vi "h5_data_2D.vi"(8 "error in (no error)":errorcluster, 11 "data":T1={"files"=[], "record"=FALSE, "save traces"=FALSE, "raw data"=[], "scope_position"=0.0, "cursors"={"A"=0.0, "B"=0.0, "C"=0.0, "D"=0.0, "E"=0.0, "F"=0.0}, "analysis_result"={"v0"=0.0, "v1"=0.0, "w0"=0.0, "w1"=0.0, "a0"=0.0, "a1"=0.0, "a2"=0.0, "f"=0.0}, "analysis_pars"=[], "func"="a0 - a1"}) -> (0 "error out":errorcluster)   [LabVIEW 2017, in "tools.lvlib"]
uses:
  tools.lvlib
  data_2D.ctl
  analysis/cursors.ctl
  analysis/analysis_result2D.ctl
  analysis/analysis_parameters.ctl
  <vilib>/UPVI/lvhdf5/dataset.llb/LVH5D Operation.ctl
  <vilib>/UPVI/lvhdf5/file.llb/LVH5F Operation.ctl
  <vilib>/UPVI/lvhdf5/dataset.llb/Simple OpenCreateReplace Dataset (Variant).vi
  <vilib>/Utility/VariantDataType/GetClusterInfo.vi
  <vilib>/Utility/VariantDataType/GetTypeInfo.vi
  <vilib>/UPVI/lvhdf5/attribute.llb/Write Multiple Attributes.vi
  <vilib>/UPVI/lvhdf5/attribute.llb/Simple H5Awrite (Variant).vi
  <vilib>/UPVI/lvhdf5/dataset.llb/H5Dwrite (Variant).vi
  <vilib>/UPVI/lvhdf5/dataset.llb/Append Element(s) to Dataset (Variant).vi
  <vilib>/UPVI/lvhdf5/dataset.llb/Simple OpenCreateReplace Dataset.xnode
  <vilib>/UPVI/lvhdf5/library.llb/HDF5 Ref.ctl
  <vilib>/UPVI/lvhdf5/attribute.llb/LVH5A Operation.ctl
  <vilib>/UPVI/lvhdf5/attribute.llb/LVH5 Write Attributes.xnode
  <vilib>/UPVI/lvhdf5/attribute.llb/Cluster to Attribute Array.xnode
  <vilib>/UPVI/lvhdf5/attribute.llb/Simple H5Awrite.xnode
  <vilib>/UPVI/lvhdf5/dataset.llb/H5Dwrite.xnode
  <vilib>/UPVI/lvhdf5/dataset.llb/Append Element(s) to Dataset.xnode
  <vilib>/Utility/VariantDataType/VariantType.lvlib
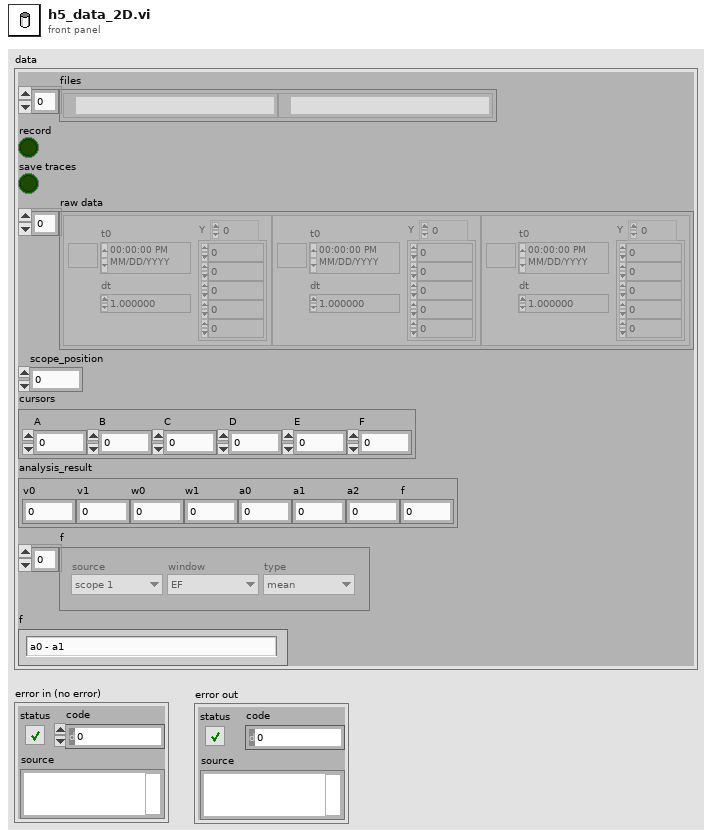
[diagram p1: front panel]
types:
  T1 = typedef "tools.lvlib/data_2D.ctl" = cluster{"files":path[], "record":bool, "save traces":bool, "raw data":waveform(dbl)[], "scope_position":dbl, "cursors":T2, "analysis_result":T3, "analysis_pars":T4[], "func":string}
  T2 = typedef "tools.lvlib/cursors.ctl" = cluster{"A":dbl, "B":dbl, "C":dbl, "D":dbl, "E":dbl, "F":dbl}
  T3 = typedef "tools.lvlib/analysis_result2D.ctl" = cluster{"v0":dbl, "v1":dbl, "w0":dbl, "w1":dbl, "a0":dbl, "a1":dbl, "a2":dbl, "f":dbl}
  T4 = typedef "tools.lvlib/analysis_parameters.ctl" = cluster{"source":enum16{"scope 0", "scope 1", "scope 2", "scope 3"}, "window":enum16{"AB", "CD", "EF"}, "type":enum16{"sum", "mean", "range"}}
  T5 = typedef "Semaphore RefNum" = refnum<k1>
  T6 = typedef "LVH5F Operation.ctl" = enum16{"open", "open or create", "create or replace", "create or replace (with confirmation)", "create", "open (read only)"}
  T7 = typedef "LVH5D Operation.ctl" = enum16{"open", "replace", "create", "open or create", "create or replace", "create or replace with confirmation"}
  T8 = typedef "HDF5 Ref.ctl" = refnum<k1>
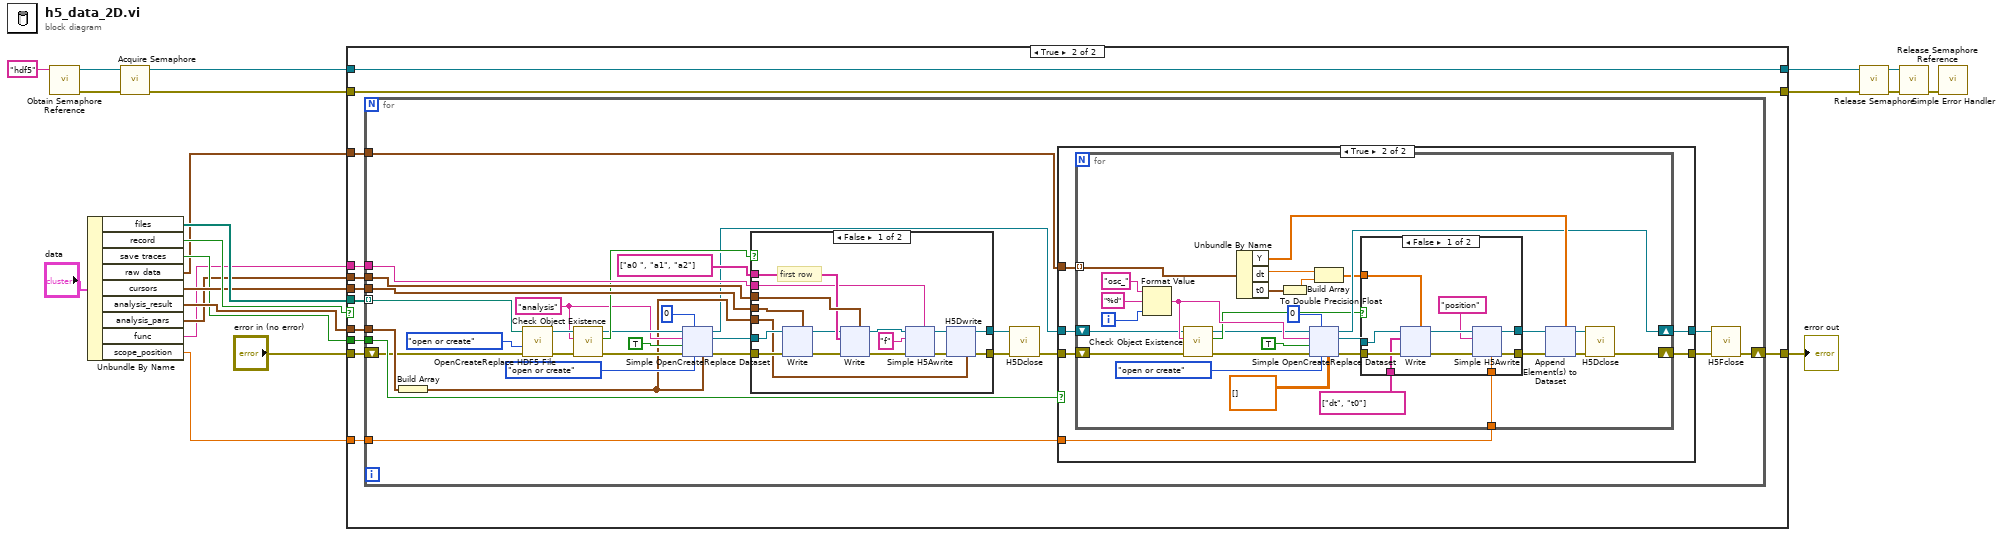
[diagram p0: block diagram]
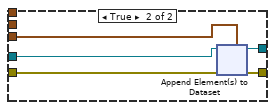
[diagram p5: hidden frame]
diagram:
  n1 = call <vilib>:"Obtain Semaphore Reference.vi"("name (unnamed)"="hdf5") -> ("error out"=w21:errorcluster, "semaphore"=w22:T5)  [unwired: 4 in, 1 out]
  n2 = Unbundle By Name("data") -> ("files"=w14:path[], "record"=w12:bool, "save traces"=w5:bool, "raw data"=w4:waveform(dbl)[], "cursors"=w7:T2, "analysis_result"=w6:T3, "analysis_pars"=w3:T4[], "func"=w2:string, "scope_position"=w1:dbl)
  n3 = call <vilib>:"Acquire Semaphore.vi"("error in (no error)"=w21, "semaphore"=w22) -> ("error out"=w11:errorcluster, "semaphore out"=w10:T5)  [unwired: 3 in, 1 out]
  n4 = case shown="True" w12 {
    tunnel: [w25 w37] -> w16
    tunnel: w14 -> [_ w36]
    tunnel: "error in (no error)" -> [w25 w35]
    tunnel: w11 -> [w24 w34]
    tunnel: w10 -> [w23 w33]
    tunnel: [w24 w34] -> w9
    tunnel: [w23 w33] -> w8
    tunnel: w7 -> [_ w32]
    tunnel: w6 -> [_ w31]
    tunnel: w5 -> [_ w30]
    tunnel: w4 -> [_ w29]
    tunnel: w3 -> [_ w28]
    tunnel: w2 -> [_ w27]
    tunnel: w1 -> [_ w26]
    frame False {
    }
    frame True {
      n5 = for {
        tunnel: w36 -> [w60] mode=indexing
        shift-right: [w46] -> w37
        shift-left: w35 -> [w59]
        tunnel: w32 -> [w67]
        tunnel: w31 -> [w66]
        tunnel: w30 -> [w65]
        tunnel: w29 -> [w64]
        tunnel: w28 -> [w62]
        tunnel: w27 -> [w61]
        tunnel: w26 -> [w38]
        w48 = "analysis" ("Dataset Path")
        n6 = Build Array(w66) -> (w45:T3[])
        n7 = call <vilib>:"OpenCreateReplace HDF5 File.vi"("error in (no error)"=w59, "function (open or create)"=LVH5F_Operation."open or create", "path"=w60) -> ("error out"=w57:errorcluster, "HDF5 Ref out"=w56:T8)  [unwired: 5 in]
        n8 = call <vilib>:"Check Object Existence.vi"("error in (no error)"=w57, "name"=w48, "HDF5 Ref"=w56) -> ("error out"=w52:errorcluster, "Exists"=w55:bool, "HDF5 Ref out"=w51:T8)  [unwired: 4 in]
        n9 = xnode "Simple OpenCreateReplace Dataset"("Compression Level (0-disabled)"=0, "Dataset Path"=w48, "HDF5 Ref"=w51, "Unlimited  dataset (F)"=TRUE, "error in (no error)"=w52, "operation"=LVH5D_Operation."open or create", "Datatype and Dataspace"=w45) -> ("HDF5 Dataset Ref out"=w47:T8, "HDF5 Ref out"=w41:T8, "error out"=w53:errorcluster)  [unwired: 1 in]
        n10 = case shown="False" w55 {
          tunnel: w53 -> [w291 w557]
          tunnel: w67 -> [w289 _]
          tunnel: string[] ["a0 ", "a1", "a2"] ("Name(s)") -> [w287 _]
          tunnel: w62 -> [w288 _]
          tunnel: w61 -> [w283 _]
          tunnel: w47 -> [w290 w558]
          tunnel: w45 -> [w276 w554]
          tunnel: [w277 w555] -> w44
          tunnel: [w278 w556] -> w43
          frame False {
            # "first row"
            n11 = xnode "Write"("HDF5 Ref"=w290, "error in (no error)"=w291, "Value(s)"=w289) -> ("HDF5 Ref out"=w281:T8, "error out"=w282:errorcluster)  [unwired: 2 in]
            n12 = xnode "Write"("HDF5 Ref"=w281, "error in (no error)"=w282, "Name(s)"=w287, "Value(s)"=w288) -> ("HDF5 Ref out"=w285:T8, "error out"=w284:errorcluster)  [unwired: 1 in]
            n13 = xnode "Simple H5Awrite"("HDF5 Ref"=w285, "Name"="f", "error in (no error)"=w284, "Value"=w283) -> ("HDF5 Ref out"=w280:T8, "error out"=w279:errorcluster)  [unwired: 1 in]
            n14 = xnode "H5Dwrite"("HDF5 Dataset Ref"=w280, "error in (no error)"=w279, "Data"=w276) -> ("HDF5 Ref out"=w277:T8, "error out"=w278:errorcluster)  [unwired: 4 in]
          }
          frame True {
            n15 = xnode "Append Element(s) to Dataset"("HDF5 Dataset Ref"=w558, "error in (no error)"=w557, "Data Element(s)"=w554) -> ("HDF5 Dataset out"=w555:T8, "error out"=w556:errorcluster)  [unwired: 1 in, 2 out]
          }
        }
        n16 = call <vilib>:"H5Dclose.vi"("error in (no error)"=w43, "HDF5 Dataset Ref"=w44) -> ("error out"=w42:errorcluster)  [unwired: 7 in]
        n17 = case shown="True" w65 {
          tunnel: [w68 w72] -> w40
          tunnel: w42 -> [w69 w74]
          tunnel: [w69 w73] -> w39
          tunnel: w64 -> [_ w75]
          tunnel: w41 -> [w68 w71]
          tunnel: w38 -> [_ w70]
          frame False {
          }
          frame True {
            n18 = for {
              tunnel: w75 -> [w77] mode=indexing
              shift-right: [w98] -> w73
              shift-left: w74 -> [w88]
              shift-right: [w89] -> w72
              shift-left: w71 -> [w85]
              tunnel: w70 -> [w76]
              i -> [w104]
              n19 = Format Value(string ("")="osc_", format string="%d", value (0)=w104) -> (output string=w86:string)
              n20 = call <vilib>:"Check Object Existence.vi"("error in (no error)"=w88, "name"=w86, "HDF5 Ref"=w85) -> ("error out"=w87:errorcluster, "Exists"=w84:bool, "HDF5 Ref out"=w83:T8)  [unwired: 4 in]
              n21 = Unbundle By Name(w77) -> ("Y"=w92:dbl[], "dt"=w81:dbl, "t0"=w82:timestamp)
              n22 = To Double Precision Float(number=w82) -> (double precision float=w80:dbl)
              n23 = xnode "Simple OpenCreateReplace Dataset"("Compression Level (0-disabled)"=0, "Dataset Path"=w86, "HDF5 Ref"=w83, "Unlimited  dataset (F)"=TRUE, "error in (no error)"=w87, "operation"=LVH5D_Operation."open or create", "Datatype and Dataspace"=dbl[][] []) -> ("HDF5 Dataset Ref out"=w95:T8, "HDF5 Ref out"=w89:T8, "error out"=w99:errorcluster)  [unwired: 1 in]
              n24 = Build Array(w81, w80) -> (w79:dbl[])
              n25 = case shown="False" w84 {
                tunnel: w95 -> [w132 w264]
                tunnel: w99 -> [w133 w263]
                tunnel: [w128 w263] -> w94
                tunnel: [w126 w264] -> w91
                tunnel: w79 -> [w131 _]
                tunnel: string[] ["dt", "t0"] ("Name(s)") -> [w130 _]
                tunnel: w76 -> [w124 _]
                frame False {
                  n26 = xnode "Write"("HDF5 Ref"=w132, "error in (no error)"=w133, "Name(s)"=w130, "Value(s)"=w131) -> ("HDF5 Ref out"=w127:T8, "error out"=w129:errorcluster)  [unwired: 1 in]
                  n27 = xnode "Simple H5Awrite"("HDF5 Ref"=w127, "Name"="position", "error in (no error)"=w129, "Value"=w124) -> ("HDF5 Ref out"=w126:T8, "error out"=w128:errorcluster)  [unwired: 1 in]
                }
                frame True {
                }
              }
              n28 = xnode "Append Element(s) to Dataset"("HDF5 Dataset Ref"=w91, "error in (no error)"=w94, "Data Element(s)"=w92) -> ("HDF5 Dataset out"=w90:T8, "error out"=w93:errorcluster)  [unwired: 1 in, 2 out]
              n29 = call <vilib>:"H5Dclose.vi"("error in (no error)"=w93, "HDF5 Dataset Ref"=w90) -> ("error out"=w98:errorcluster)  [unwired: 7 in]
            }
          }
        }
        n30 = call <vilib>:"H5Fclose.vi"("error in (no error)"=w39, "HDF5 Ref"=w40) -> ("error out"=w46:errorcluster)  [unwired: 7 in]
      }
    }
  }
  "error out" <- w16
  n31 = call <vilib>:"Release Semaphore.vi"("error in (no error)"=w9, "semaphore"=w8) -> ("error out"=w19:errorcluster, "semaphore out"=w18:T5)  [unwired: 4 in]
  n32 = call <vilib>:"Release Semaphore Reference.vi"("error in (no error)"=w19, "semaphore"=w18) -> ("error out"=w17:errorcluster)  [unwired: 8 in, 1 out]
  n33 = call <vilib>:"Simple Error Handler.vi"("error in (no error)"=w17) -> ()  [unwired: 4 in, 5 out]
